vi "getFPGA.vi"(11 "ModbusSubnetETxDataFIFO in":refnum<class "ModbusSubnetETxDataFIFO.lvclass">) -> (2 "FPGA":refnum<class "FPGA.lvclass">, 3 "ModbusSubnetETxDataFIFO out":refnum<class "ModbusSubnetETxDataFIFO.lvclass">)   [LabVIEW 2016, in "ModbusSubnetETxDataFIFO.lvclass"]
uses:
  ModbusSubnetETxDataFIFO.lvclass
  FPGA/FPGA.lvclass
  ModbusSubnetETxDataFIFO.lvclass/ModbusSubnetETxDataFIFO.ctl
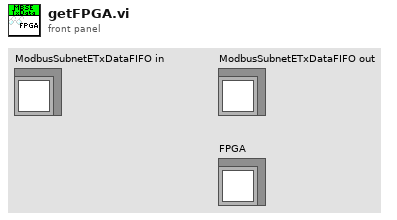
[diagram p1: front panel]
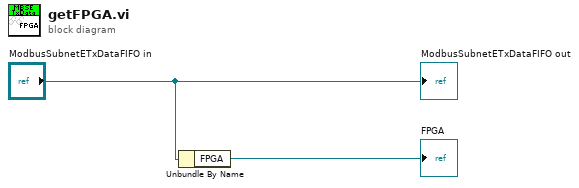
[diagram p0: block diagram]
diagram:
  n1 = Unbundle By Name("ModbusSubnetETxDataFIFO in") -> ("FPGA"=→"FPGA":refnum<class "FPGA.lvclass">)
  "ModbusSubnetETxDataFIFO out" <- "ModbusSubnetETxDataFIFO in"
